vi "Close.vi"(8 "error in (no error)":errorcluster, 11 "Generic Digital Multi Meter in":refnum<class "Generic Digital Multi Meter.lvclass">) -> (0 "error out":errorcluster, 3 "Generic Digital Multi Meter out":refnum<class "Generic Digital Multi Meter.lvclass">)   [LabVIEW 2014, in "Generic Digital Multi Meter.lvlib" / "Generic Digital Multi Meter.lvclass"]
uses:
  Generic Digital Multi Meter.lvclass
  Abstract Sensor/Abstract Sensor.lvclass
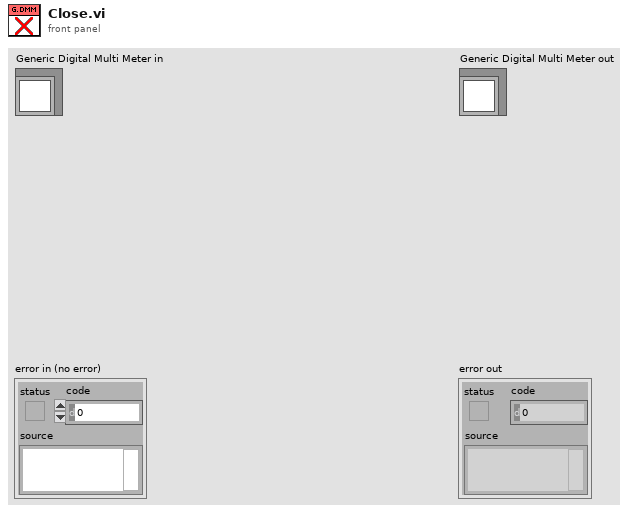
[diagram p1: front panel]
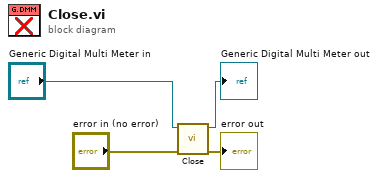
[diagram p0: block diagram]
diagram:
  n1 = call-parent "Close.vi"("error in (no error)"="error in (no error)", "Abstract Sensor in"="Generic Digital Multi Meter in") -> ("error out"=→"error out":errorcluster, "Abstract Sensor out"=→"Generic Digital Multi Meter out":refnum<class "Generic Digital Multi Meter.lvclass">)  [unwired: 8 in]
